vi "SetTriggerOutput.vi"(8 "Error In":errorcluster, 10 "Trigger Output":T1, 11 "Keithley 6485 In":refnum<visa-resource-name>) -> (0 "Error Out":errorcluster, 3 "Keithley 6485 Out":refnum<visa-resource-name>)   [LabVIEW 2012, in "Keithley-6485.lvlib"]
uses:
  Keithley-6485.lvlib
  Controls/TriggerOutput.ctl
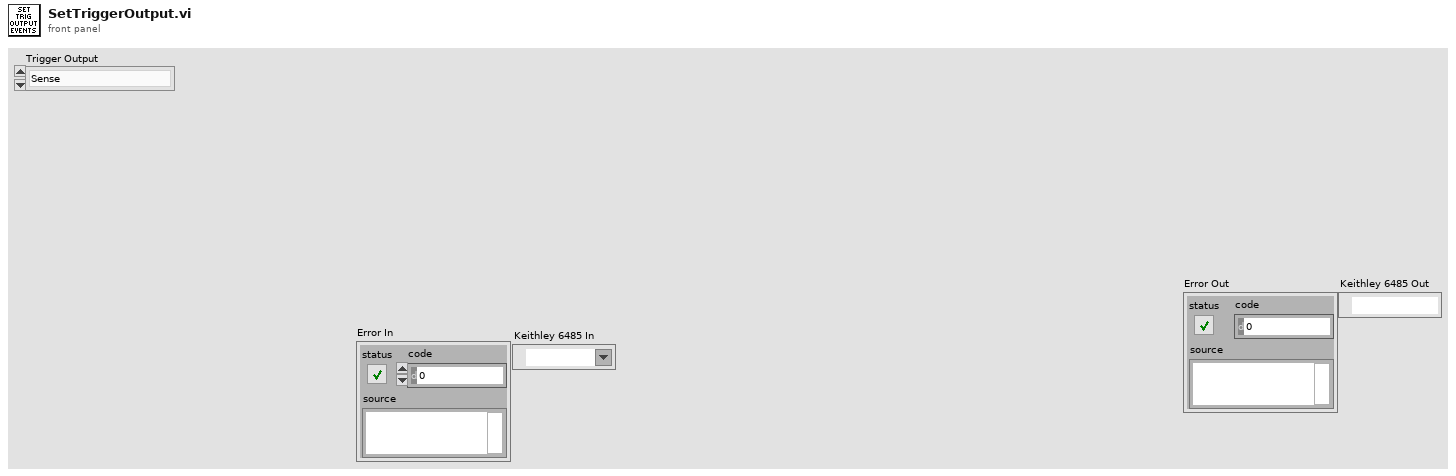
[diagram p1: front panel]
types:
  T1 = typedef "Keithley-6485.lvlib/TriggerOutput.ctl" = enum16{"Sense", "None"}
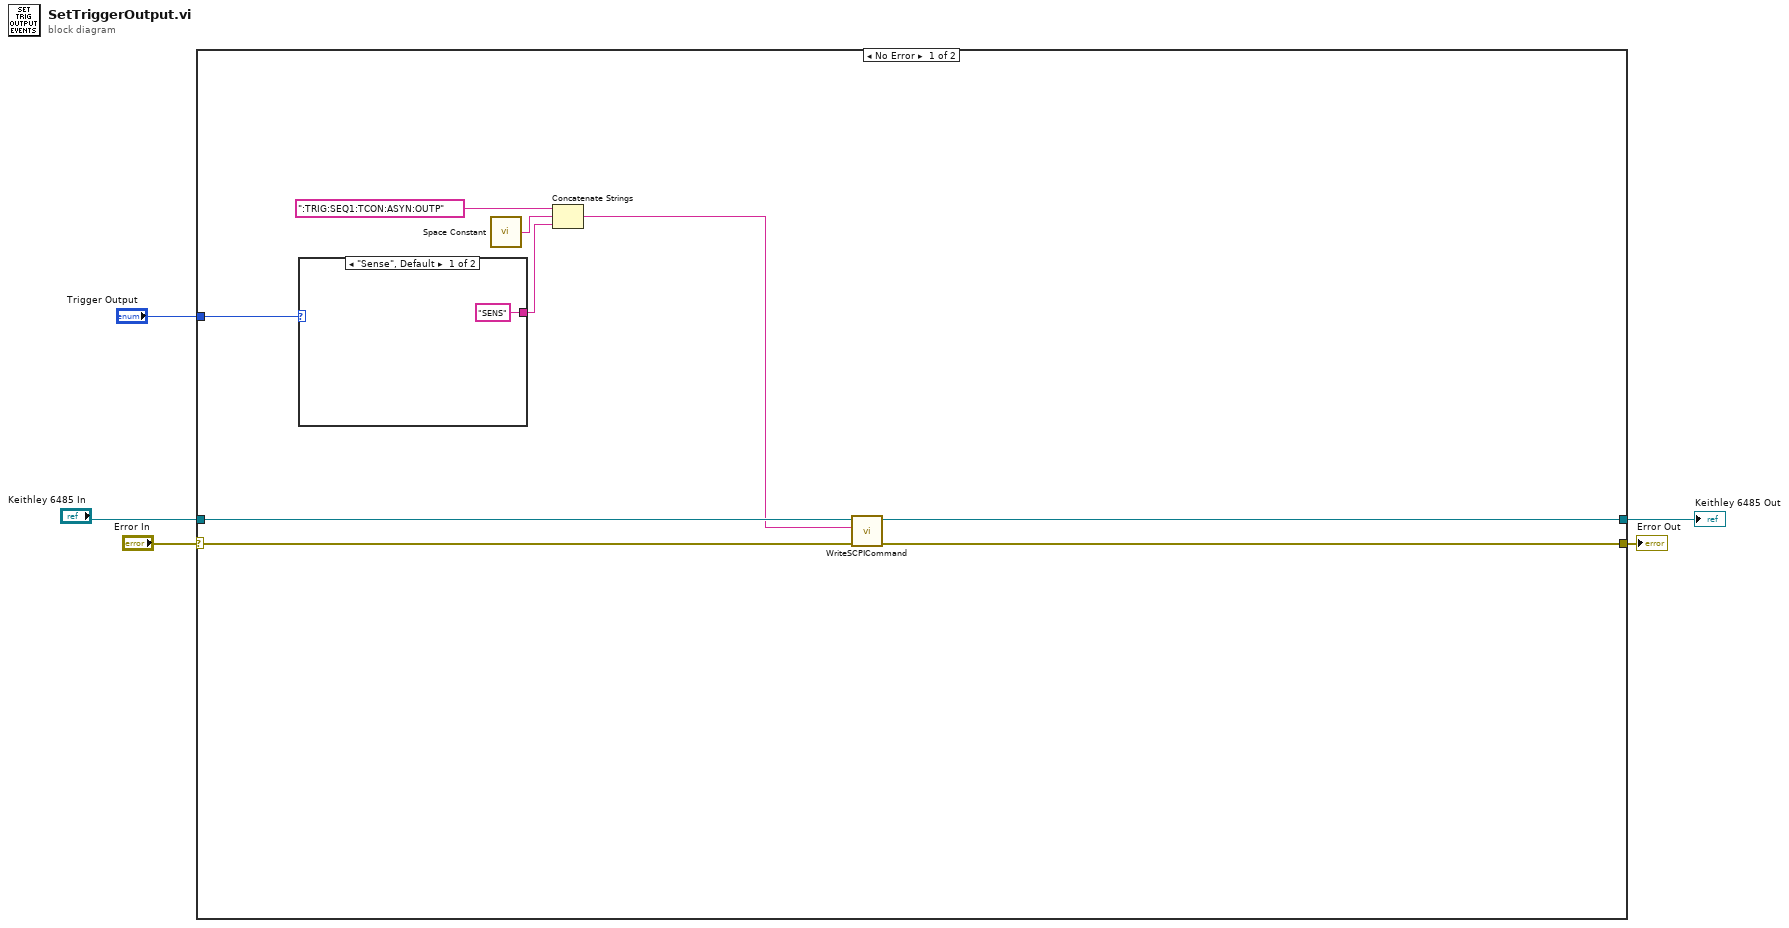
[diagram p0: block diagram]
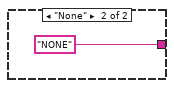
[diagram p2: hidden frame]
diagram:
  n1 = case shown="No Error" "Error In" {
    selector: "Error In" -> [w14 w17]
    tunnel: [w13 w17] -> w4
    tunnel: [w12 w18] -> w3
    tunnel: "Keithley 6485 In" -> [w11 w18]
    tunnel: "Trigger Output" -> [w7 _]
    frame No Error {
      n2 = case shown="\"Sense\", Default" w7 {
        tunnel: ["SENS" "NONE"] -> w6
        frame "Sense", Default {
        }
        frame "None" {
        }
      }
      n3 = call <vilib>:"Space Constant.vi"() -> ("String"=w9:string)
      n4 = Concatenate Strings(":TRIG:SEQ1:TCON:ASYN:OUTP", w9, w6) -> (w8:string)
      n5 = call "WriteSCPICommand.vi"("Error In"=w14, "SCPI Command"=w8, "Keithley 6482 In"=w11) -> ("Error Out"=w13:errorcluster, "Keithley 6482 Out"=w12:refnum<visa-resource-name>)  [unwired: 7 in]
    }
    frame Error {
    }
  }
  "Error Out" <- w4
  "Keithley 6485 Out" <- w3
